vi "Read.vi"(8 "error in (no error)":errorcluster, 11 "Numeric in":refnum<class "Const_U64.lvclass">) -> (0 "error out":errorcluster, 2 "Numeric":T1, 3 "Numeric out":refnum<class "Const_U64.lvclass">)   [LabVIEW 2021, in "Const_U64.lvclass"]
uses:
  Const_U64.lvclass
  Type.ctl
  Const_U64.lvclass/Const_U64.ctl
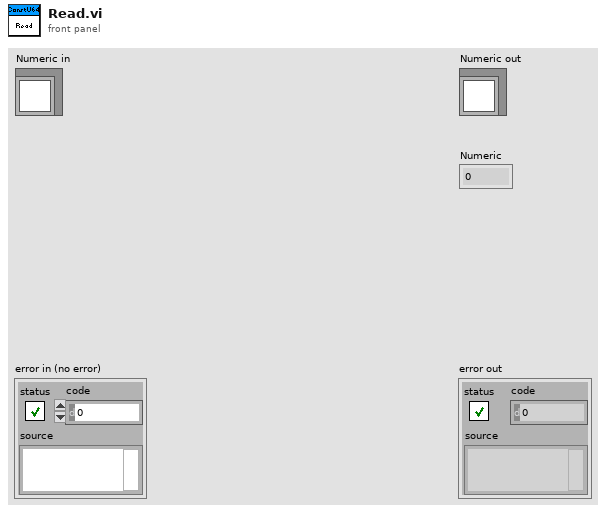
[diagram p1: front panel]
types:
  T1 = typedef "Const_U64.lvclass/Type.ctl" = u64
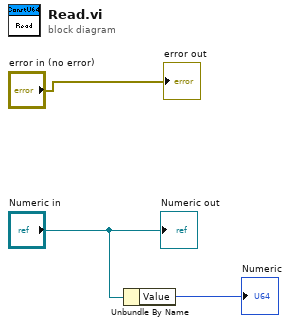
[diagram p0: block diagram]
diagram:
  n1 = Unbundle By Name("Numeric in") -> ("Value"=→"Numeric":T1)
  "error out" <- "error in (no error)"
  "Numeric out" <- "Numeric in"
